vi "Read WiFi RSSI.vi"() -> (0 "error out":errorcluster)   [LabVIEW 2020]
panel:
  out "Error String":string
  out "Raw Value":dbl format="%.6f"
  in  "Name":string="WIFI_RSSI"
  out "ConnectionType Out":i32
  out "DeviceType Out":i32
  in  "Identifier":string="LJM_idANY"
  in  "ConnectionType":string="LJM_ctANY"
  in  "DeviceType":string="LJM_dtANY"
  # "RSSI is only updated on WiFi communication, so\nif this VI is reading RSSI over USB or Ethernet you\nwill get the value as of the last WiFi communication\nthat occurred."
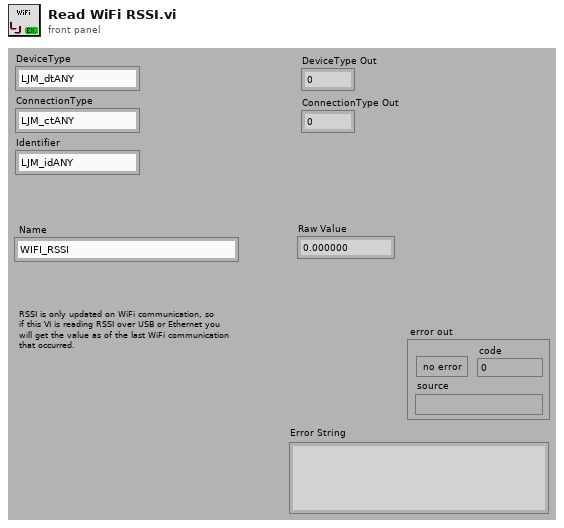
[diagram p1: front panel]
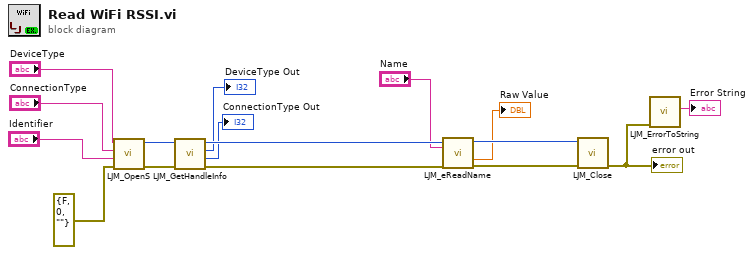
[diagram p0: block diagram]
diagram:
  n1 = call "LJM_OpenS.vi"("error in"=errorcluster {"status"=FALSE, "code"=0, "source"=""} ("error in (no error)"), "Identifier"="Identifier", "ConnectionType"="ConnectionType", "DeviceType"="DeviceType") -> ("error out"=w14:errorcluster, "Handle"=w12:i32)  [unwired: 6 in]
  n2 = call "LJM_GetHandleInfo.vi"("error in"=w14, "Handle In"=w12) -> ("error out"=w13:errorcluster, "ConnectionType"=→"ConnectionType Out":i32, "DeviceType"=→"DeviceType Out":i32, "Handle Out"=w11:i32)  [unwired: 2 in, 4 out]
  n3 = call "LJM_eReadName.vi"("Handle In"=w11, "Name"="Name", "error in"=w13) -> ("Handle Out"=w10:i32, "Value"=→"Raw Value":dbl, "error out"=w15:errorcluster)  [unwired: 10 in]
  n4 = call "LJM_Close.vi"("error in"=w15, "Handle"=w10) -> ("error out"=w3:errorcluster)  [unwired: 9 in]
  "error out" <- w3
  n5 = call "LJM_ErrorToString.vi"("error in"=w3) -> ("String"=→"Error String":string)  [unwired: 10 in]
